vi "Initialize.vi"(8 "error in (no error)":errorcluster, 11 "RS232 in":refnum<class "RS-xxx.lvclass">) -> (0 "error out":errorcluster, 3 "RS232 out":refnum<class "RS-xxx.lvclass">)   [LabVIEW 2013, in "Protocol Classes.lvlib" / "RS-xxx.lvclass"]
uses:
  RS-xxx.lvclass
  Protocol Parent/Protocol Parent.lvclass
  RS-xxx.lvclass/RS-xxx.ctl
  <vilib>/Instr/_visa.llb/VISA Configure Serial Port (Instr).vi
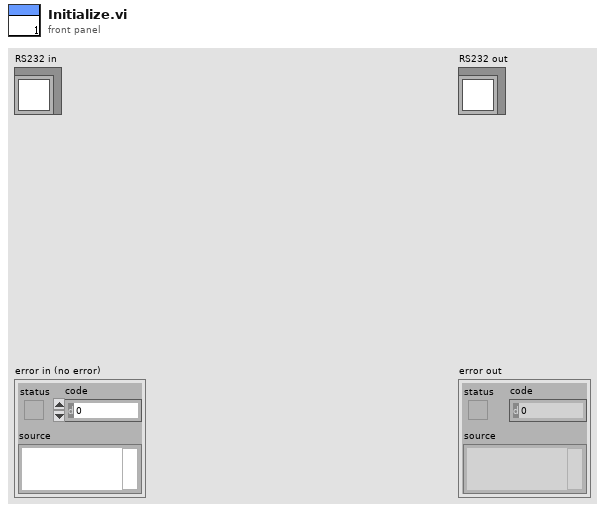
[diagram p1: front panel]
types:
  T1 = cluster{"Port":string, "Baud Rate":u32, "Data Bits":u16, "Parity":enum16{"None", "Odd", "Even", "Mark", "Space"}, "Stop Bits":u16, "Flow Control":u16, "XON":enum16{"NUL", "SOH", "STX", "ETX", "EOT", "ENQ", "ACK", "BEL", "BS", "HT", "LF", "VT", "FF", "CR", "SO", "SI", "DLE", "DC1", "DC2", "DC3", "DC4", "NAK", "SYN", "ETB", "CAN", "EM", "SUB", "ESC", "FS", "GS", "RS", "US", "SP", "!", "\"", "#", "$", "%", "&", "'", "(", ")", "*", "+", ",", "- (-)", ".", "/", "0", "1", "2", "3", "4", "5", "6", "7", "8", "9", ":", ";", "<", "=", ">", "?", "@", "A", "B", "C", "D", "E", "F", "G", "H", "I", "J", "K", "L", "M", "N", "O", "P", "Q", "R", "S", "T", "U", "V", "W", "X", "Y", "Z", "[", "\\", "]", "^", "_", "`", "a", "b", "c", "d", "e", "f", "g", "h", "i", "j", "k", "l", "m", "n", "o", "p", "q", "r", "s", "t", "u", "v", "w", "x", "y", "z", "{", "|", "}", "~"}, "XOFF":enum16{"NUL", "SOH", "STX", "ETX", "EOT", "ENQ", "ACK", "BEL", "BS", "HT", "LF", "VT", "FF", "CR", "SO", "SI", "DLE", "DC1", "DC2", "DC3", "DC4", "NAK", "SYN", "ETB", "CAN", "EM", "SUB", "ESC", "FS", "GS", "RS", "US", "SP", "!", "\"", "#", "$", "%", "&", "'", "(", ")", "*", "+", ",", "- (-)", ".", "/", "0", "1", "2", "3", "4", "5", "6", "7", "8", "9", ":", ";", "<", "=", ">", "?", "@", "A", "B", "C", "D", "E", "F", "G", "H", "I", "J", "K", "L", "M", "N", "O", "P", "Q", "R", "S", "T", "U", "V", "W", "X", "Y", "Z", "[", "\\", "]", "^", "_", "`", "a", "b", "c", "d", "e", "f", "g", "h", "i", "j", "k", "l", "m", "n", "o", "p", "q", "r", "s", "t", "u", "v", "w", "x", "y", "z", "{", "|", "}", "~"}, "End Read on Termination Character":bool, "End Write on Termination Character":bool, "Termination Character":u8}
  T2 = enum16{"NUL", "SOH", "STX", "ETX", "EOT", "ENQ", "ACK", "BEL", "BS", "HT", "LF", "VT", "FF", "CR", "SO", "SI", "DLE", "DC1", "DC2", "DC3", "DC4", "NAK", "SYN", "ETB", "CAN", "EM", "SUB", "ESC", "FS", "GS", "RS", "US", "SP", "!", "\"", "#", "$", "%", "&", "'", "(", ")", "*", "+", ",", "- (-)", ".", "/", "0", "1", "2", "3", "4", "5", "6", "7", "8", "9", ":", ";", "<", "=", ">", "?", "@", "A", "B", "C", "D", "E", "F", "G", "H", "I", "J", "K", "L", "M", "N", "O", "P", "Q", "R", "S", "T", "U", "V", "W", "X", "Y", "Z", "[", "\\", "]", "^", "_", "`", "a", "b", "c", "d", "e", "f", "g", "h", "i", "j", "k", "l", "m", "n", "o", "p", "q", "r", "s", "t", "u", "v", "w", "x", "y", "z", "{", "|", "}", "~"}
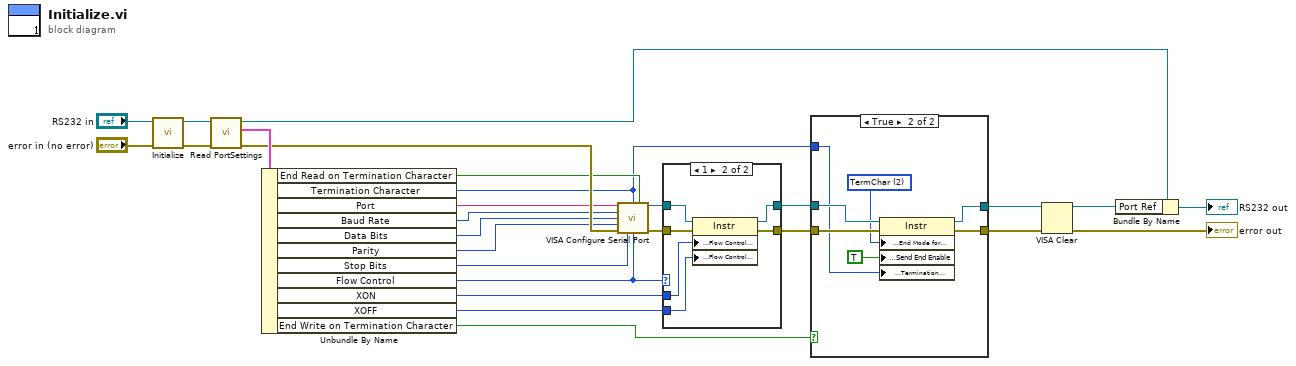
[diagram p0: block diagram]
diagram:
  n1 = call-parent "Initialize.vi"("error in (no error)"="error in (no error)", "Protocol Parent in"="RS232 in") -> ("error out"=w24:errorcluster, "Protocol Parent out"=w25:refnum<class "RS-xxx.lvclass">)  [unwired: 8 in]
  n2 = call "Read PortSettings.vi"("error in (no error)"=w24, "RS232 in"=w25) -> ("error out"=w22:errorcluster, "Cluster"=w23:T1, "RS232 out"=w6:refnum<class "RS-xxx.lvclass">)  [unwired: 7 in]
  n3 = Unbundle By Name(w23) -> ("End Read on Termination Character"=w14:bool, "Termination Character"=w7:u8, "Port"=w21:string, "Baud Rate"=w20:u32, "Data Bits"=w19:u16, "Parity"=w18:enum16{"None", "Odd", "Even", "Mark", "Space"}, "Stop Bits"=w17:u16, "Flow Control"=w12:u16, "XON"=w13:T2, "XOFF"=w11:T2, "End Write on Termination Character"=w8:bool)
  n4 = call-poly "VISA Configure Serial Port"("VISA resource name"=w21, "termination char\n(0xA = '\\n' = LF)"=w7, "Enable Termination\nChar (T)"=w14, "baud rate (9600)"=w20, "data bits (8)"=w19, "parity (0:none)"=w18, "error in (no error)"=w22, "stop bits (10: 1 bit)"=w17, "flow control (0:none)"=w12) -> ("VISA resource name out"=w9:refnum<visa-resource-name>, "error out"=w10:errorcluster)  [unwired: 5 in]
  n5 = case shown="1" w12 {
    tunnel: [w28 w35] -> w15
    tunnel: [w29 w34] -> w16
    tunnel: w10 -> [w28 w33]
    tunnel: w9 -> [w29 w32]
    tunnel: w13 -> [_ w31]
    tunnel: w11 -> [_ w30]
    frame Default {
    }
    frame 1 {
      n6 = property class="Instr"(reference=w32, error in=w33, "Serial Settings:Flow Control XON Character"=w31, "Serial Settings:Flow Control XOFF Character"=w30) -> (reference out=w34:refnum<visa-resource-name>, error out=w35:errorcluster)
    }
  }
  n7 = case shown="True" w8 {
    tunnel: w16 -> [w36 w44]
    tunnel: w15 -> [w37 w43]
    tunnel: [w36 w42] -> w3
    tunnel: [w37 w41] -> w2
    tunnel: w7 -> [_ w39]
    frame False {
    }
    frame True {
      w40 = u16 2 items=["None", "LastBit", "TermChar", "Break"] ("Serial Settings:Serial End Mode for Writes")
      n8 = property class="Instr"(reference=w44, error in=w43, "Serial Settings:End Mode for Writes"=w40, "Message Based Settings:Send End Enable"=TRUE, "Message Based Settings:Termination Character"=w39) -> (reference out=w42:refnum<visa-resource-name>, error out=w41:errorcluster)
    }
  }
  n9 = VISA Clear(VISA resource name=w3, error in (no error)=w2) -> (VISA resource name out=w4:refnum<visa-resource-name>, error out=→"error out":errorcluster)
  n10 = Bundle By Name(cluster=w6, "Port Ref"=w4) -> (→"RS232 out":refnum<class "RS-xxx.lvclass">)
